vi "hmi3.vi"() -> ()   [LabVIEW 2017]
doc: "Demonstrates how to write and receive CAN frames via the Network Interface on the same port. \n\nTo write and receive frames via the Network Interface:\n- select the CAN Network Interface (i.e. CAN0, CAN1, etc.)\n- select the Baud Rate\n- run the VI\n- press the write button to write frames to the can bus\n\nEnable RTR Button to send a Remote Transmission Request or to simply send an empty Frame to request an Answer Frame from a connected device.\n\nEnable Extended Button to write extended Identifier Format. This is done by setting the 30th bit to enable extended format with the driver."
uses:
  <vilib>/nican/nican.llb/ncNetAttr.ctl
panel:
  out "Data":u8[](array[numeric])
  out "Heartbeat":u16 format="%04x"
  in  "interface":string(combo)="CAN0" caption="Interface"
  in  "shutdown":bool
  # "PRESS AND HOLD"
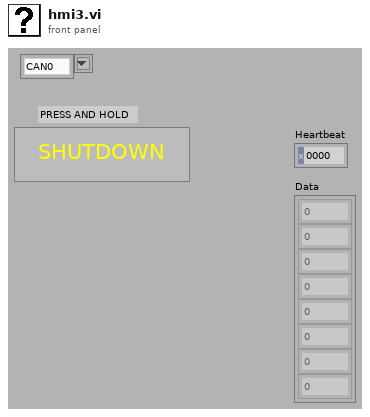
[diagram p1: front panel]
types:
  T1 = typedef "ncNetAttr.ctl" = cluster{"Start On Open":enum32{"FALSE", "TRUE"}, "Baud Rate":u32, "Read Queue Length":u32, "Write Queue Length":u32, "Standard Comparator":u32, "Standard Mask":u32, "Extended Comparator":u32, "Extended Mask":u32}
  T2 = typedef "xobjhandle.ctl" = u32
  T3 = typedef "CanFrameTimed.ctl" = cluster{"Timestamp":dbl, "ArbitrationId":u32, "IsRemote":u8, "DataLength":u8, "Data":u8[]}
  T4 = cluster{dbl, u32, "IsRemote":u8, "DataLength":u8, u8[]}
  T5 = cluster{dbl, u32, "IsRemote":u8, "DataLength":u8, u8[]}[]
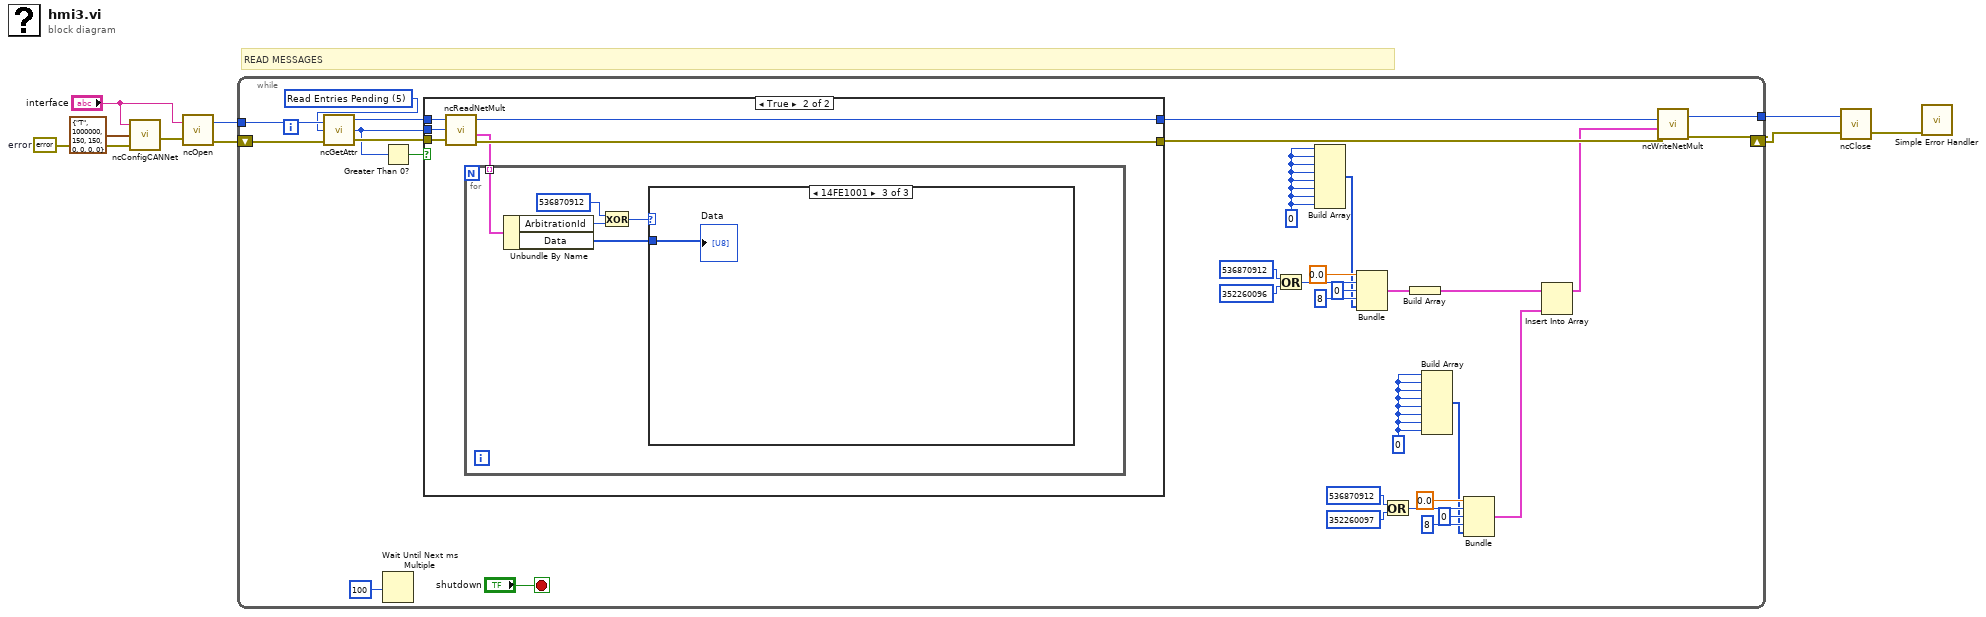
[diagram p0: block diagram]
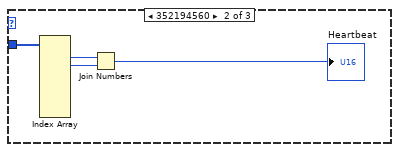
[diagram p4: hidden frame]
diagram:
  w5 = errorcluster {"status"=FALSE, "code"=0, "source"=""}  # error
  # "READ MESSAGES"
  n1 = call <vilib>:"ncConfigCANNet.vi"("Error in"=w5, "CAN Network Interface Config"=T1 {"Start On Open"=enum."TRUE", "Baud Rate"=1000000, "Read Queue Length"=150, "Write Queue Length"=150, "Standard Comparator"=0, "Standard Mask"=0, "Extended Comparator"=0, "Extended Mask"=0}, "ObjName"="interface") -> ("Error out"=w6:errorcluster)  [unwired: 2 in]
  n2 = call <vilib>:"ncOpen.vi"("Error in"=w6, "ObjName"="interface") -> ("Error out"=w9:errorcluster, "ObjHandle out"=w7:T2)
  n3 = while {
    tunnel: w7 -> [w36]
    tunnel: [w41] -> w2
    shift-right: [w42] -> w1
    shift-left: w9 -> [w35]
    stop <- "shutdown" stop-if-true
    w12 = u8 0
    w20 = u8 0
    w32 = u32 5 items=["(reserved)", "Protocol Version", "Software Version", "Object State", "(reserved)", "Read Entries Pending", "Write Entries Pending", "ReadMult Size for Notification", "Listen Only?", "Self Reception?", "Transmit Error Counter", "Receive Error Counter", "Single Shot Transmit?", "Series 2 Filter Mode", "Series 2 Mask", "Series 2 Comparator", "Serial Number", "Form Factor", "Series", "Transceiver Type", "Interface Number", "Series 2 Error/Arb Capture", "Transceiver Mode", "Transceiver External Outputs", "Transceiver External Inputs", "Start Trigger Behavior", "Log Comm Warnings", "User RTSI Frame", "Transmit Mode", "Log Start Trigger?", "Timestamp Format", "Master Timebase Rate", "Virtual Bus Timing"] ("AttrId")
    n4 = call <vilib>:"ncGetAttr.vi"("Error in"=w35, "AttrId"=w32, "ObjHandle in"=w36) -> ("Error out"=w40:errorcluster, "AttrValue"=w37:u32, "ObjHandle out"=w39:T2)
    n5 = Greater Than 0?(x=w37) -> (x > 0?=w38:bool)
    n6 = Wait Until Next ms Multiple(millisecond multiple=u32 100) -> ()  [unwired: 1 out]
    n7 = case shown="True" w38 {
      tunnel: [w43 w50] -> w33
      tunnel: [w44 w49] -> w34
      tunnel: w37 -> [_ w48]
      tunnel: w40 -> [w43 w47]
      tunnel: w39 -> [w44 w46]
      frame False {
      }
      frame True {
        n8 = call <vilib>:"ncReadNetMult.vi"("ObjHandle in"=w46, "Requested Number of Frames"=w48, "Error in"=w47) -> ("ObjHandle out"=w49:T2, "Data"=w45:T3[], "Error out"=w50:errorcluster)  [unwired: 1 out]
        n9 = for {
          tunnel: w45 -> [w55] mode=indexing
          n10 = Unbundle By Name(w55) -> ("ArbitrationId"=w53:u32, "Data"=w51:u8[])
          n11 = Exclusive Or(1:w53, 2:u32 536870912 ("y")) -> (0:w52:u32)
          n12 = case shown="14FE1001" w52 {
            tunnel: w51 -> [_ w59 w60]
            frame Default {
            }
            frame 352194560 {
              n13 = Index Array(array=w59) -> (element #1=w57:u8, element #2=w58:u8)  [unwired: 8 in, 6 out]
              n14 = Join Numbers(hi=w57, lo=w58) -> ((hi.lo)=→"Heartbeat":u16)
            }
            frame 352194561 {
              "Data" <- w60
            }
          }
        }
      }
    }
    n15 = Or(x=u32 536870912 ("y"), y=u32 352260096) -> (x .or. y?=w18:u32)
    n16 = Build Array(w12, w12, w12, w12, w12, w12, w12, w12) -> (w14:u8[])
    n17 = Bundle(0.0, w18, "IsRemote"=u8 0, "DataLength"=u8 8, w14) -> (w11:T4)  [unwired: 1 in]
    n18 = Or(x=u32 536870912 ("y"), y=u32 352260097) -> (x .or. y?=w27:u32)
    n19 = Build Array(w11) -> (w10:T5)
    n20 = Build Array(w20, w20, w20, w20, w20, w20, w20, w20) -> (w23:u8[])
    n21 = Bundle(0.0, w27, "IsRemote"=u8 0, "DataLength"=u8 8, w23) -> (w29:T4)  [unwired: 1 in]
    n22 = Insert Into Array(array=w10, new element=w29) -> (w21:T5)  [unwired: 1 in]
    n23 = call <vilib>:"ncWriteNetMult.vi"("Error in"=w33, "Data"=w21, "ObjHandle in"=w34) -> ("Error out"=w42:errorcluster, "ObjHandle out"=w41:T2)  [unwired: 7 in]
  }
  n24 = call <vilib>:"ncClose.vi"("Error in"=w1, "ObjHandle in"=w2) -> ("Error out"=w3:errorcluster)  [unwired: 1 in]
  n25 = call <vilib>:"Simple Error Handler.vi"("error in (no error)"=w3) -> ()  [unwired: 4 in, 5 out]
